vi "Get Velocity.vi"(8 "error in (no error)":errorcluster, 11 "NI_Robotics_KUKA youBot Gripper Motor in":refnum<class "NI_Robotics_KUKA youBot Gripper Motor.lvclass">) -> (0 "error out":errorcluster, 2 "ccw velocity (rpm)":dbl, 3 "NI_Robotics_KUKA youBot Gripper Motor out":refnum<class "NI_Robotics_KUKA youBot Gripper Motor.lvclass">)   [LabVIEW 2017, in "NI_Robotics_KUKA youBot Host.lvlib" / "NI_Robotics_KUKA youBot Gripper Motor.lvclass"]
uses:
  <vilib>/robotics/KUKA youBot/Motor/Gripper Motor/NI_Robotics_KUKA youBot Gripper Motor.lvclass
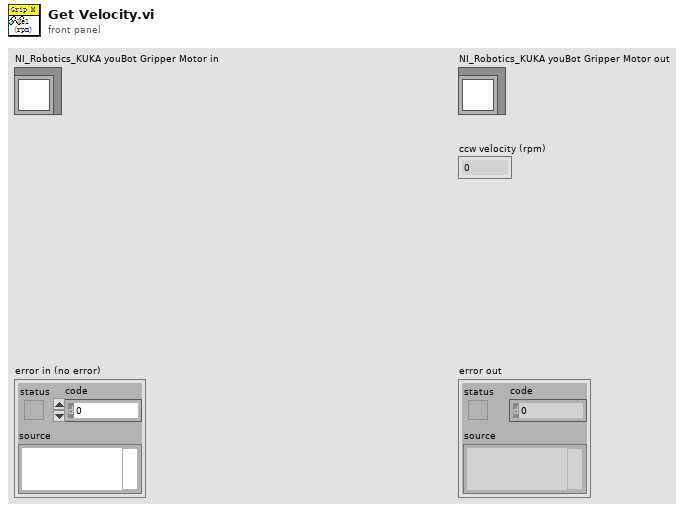
[diagram p1: front panel]
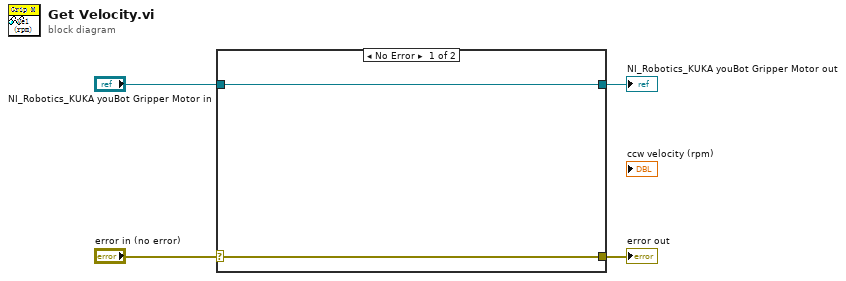
[diagram p0: block diagram]
diagram:
  n1 = case shown="No Error" "error in (no error)" {
    selector: "error in (no error)" -> [w6 w7]
    tunnel: [w6 w7] -> w3
    tunnel: [w5 w8] -> w1
    tunnel: "NI_Robotics_KUKA youBot Gripper Motor in" -> [w5 w8]
    frame No Error {
    }
    frame Error {
    }
  }
  "error out" <- w3
  "NI_Robotics_KUKA youBot Gripper Motor out" <- w1
